vi "GetPositionDegreesSpeed.vi"(0 "StepMotor in":refnum<class "StepMotor.lvclass">, 2 "Редукция":dbl, 3 "Разрешение энкодера":dbl, 5 "error in (no error)":errorcluster) -> (14 "StepMotor out":refnum<class "StepMotor.lvclass">, 16 "Значение":dbl, 17 "+360 -360":bool, 18 "+ 0 -":bool, 19 "error out":errorcluster)   [LabVIEW 2010, in "StepMotor.lvclass"]
doc: "Подпрограмма получает значение энкодера СПШ и в зависимости от редукции и разрешения энкодера пересчитывает в градусы, диапазон значений энкодера варьируется от \"+\" к \"-\" значениям, это значит, что двигатель делает два оборота в левую сторону отрицательные значения и в правую сторону положительные значения. \n\n- Выходной параметр \"+ 0 -\" фиксирует переход от положительного диапазона к отрицательному диапазону или на оборот. \n\n- Выходной параметр \"+360 -360\" фиксирует состояния выхода значения энкодера за диапазон допустимый, как положительных значений, так и отрицательные значений, допустимый диапазон рассчитывается в зависимости от входных параметров \"Редукция\" и \"Разрешение энкодера\". Этот параметр необходим для обнуления внутренних переменных СПШ \"Текущая позиция\" и \"Заданная позиция\" функцией PCUR внутреннего ПЛК СПШ путём вызова из банка программ программу, в которой эта функция прописана\nПример:\n X=W //Сохраняем текущую скорость в переменную X\n W=0,A=10000 //Обнуляем скорость с ускорением 10000\n P=P,A=10000 // Заданной позиции присваиваем Текущую позицию\n PCUR=0 // Обнуляем текущую позицию и заданную позицию\n W=X // Присваиваем скорости значение сохранённое в переменной X\n HALT // Конец программы\n\nЭто позволяет контролировать много оборотов вала редуктора или двигателя при вращении в одну сторону, так как значение энкодера СПШ инкрементируются до ограниченного размера переменной в памяти контроллера ПЛК СПШ и ограничиваются диапазоном от 2147483648(параметр ПЛК ip14 прав.) до -2147483648(параметр ПЛК ip13 лев.) .\n\n-Выходной параметр \"Значение\" возвращает значение энкодера переведённое в градусы"
uses:
  StepMotor.lvclass
panel:
  out "Waveform Chart":dynamicdata(graph)
  out "РазностьТекущПреды":dbl
  out "RawValue":dbl
  out "МножПриведШкалы360":dbl
  out "КолИмпулОборот":dbl
  out "Текущая позиция":dbl
  out "Предыдущая позиция":dbl
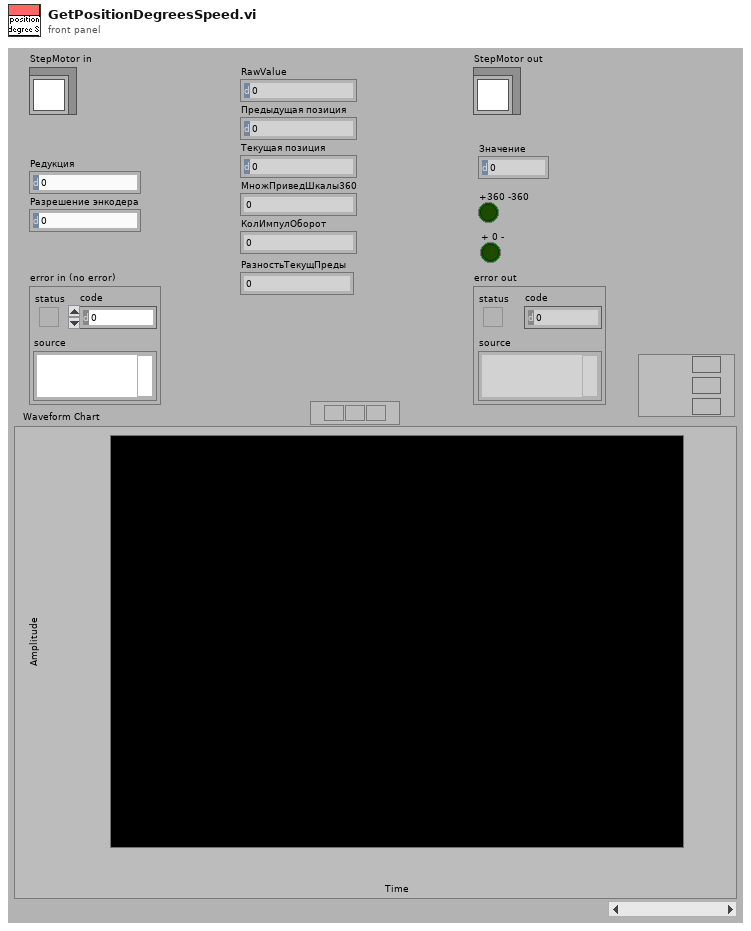
[diagram p1: front panel]
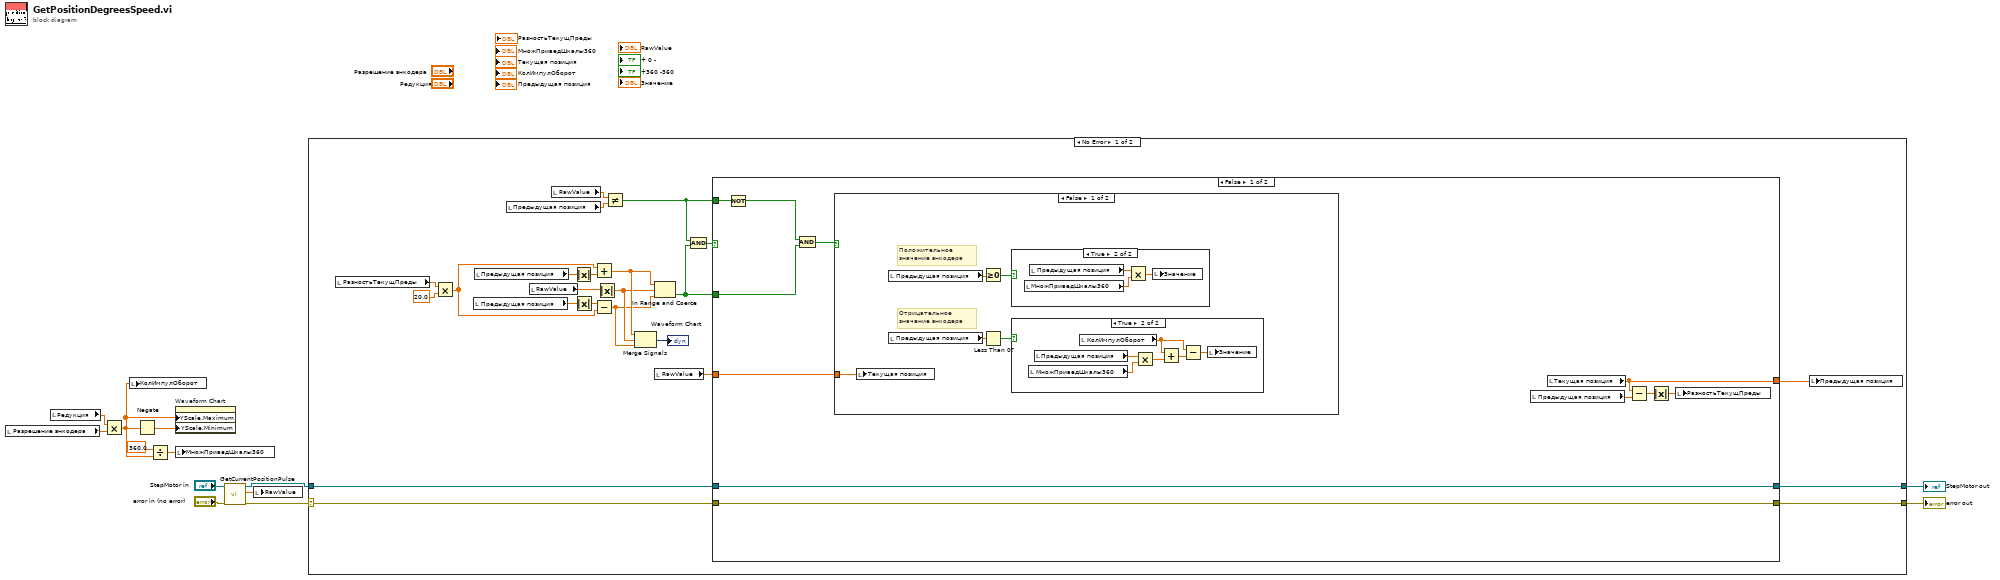
[diagram p0: block diagram]
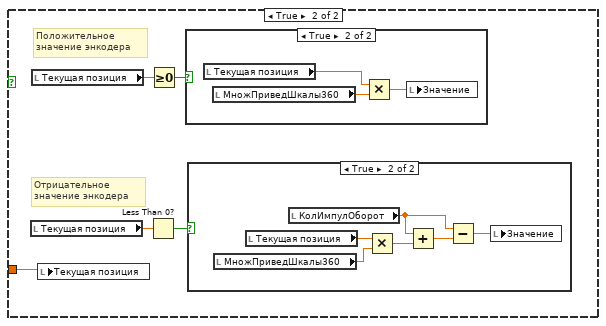
[diagram p4: hidden frame]
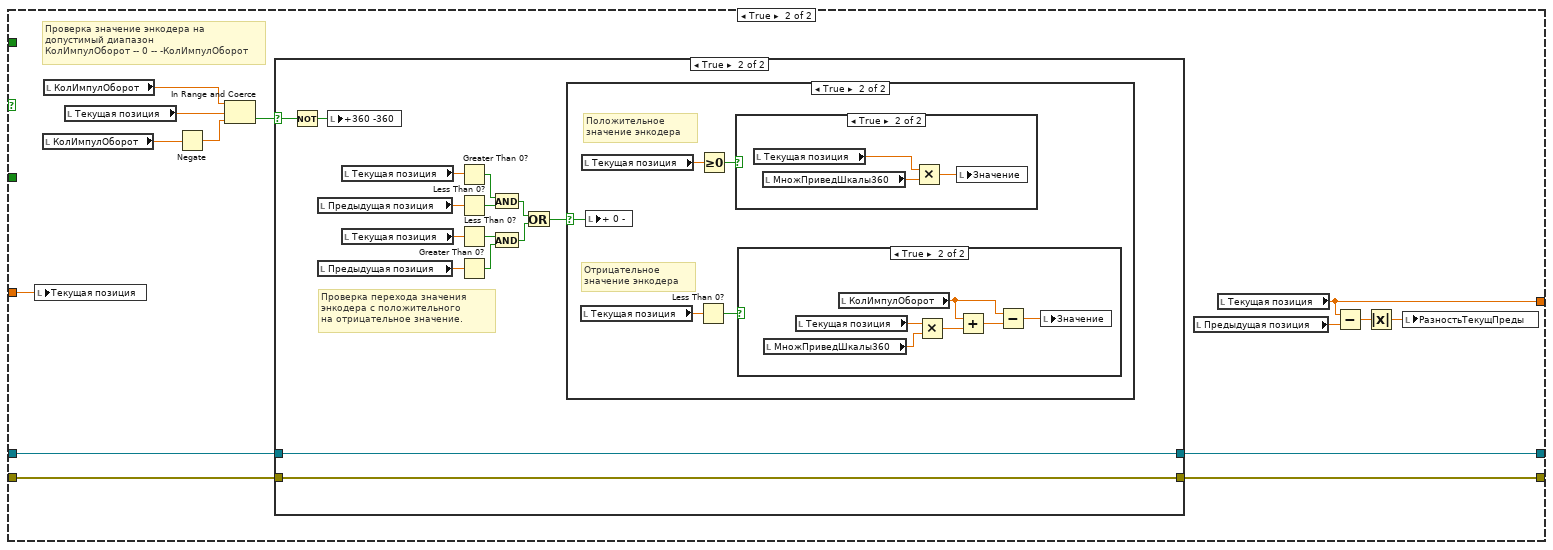
[diagram p7: hidden frame]
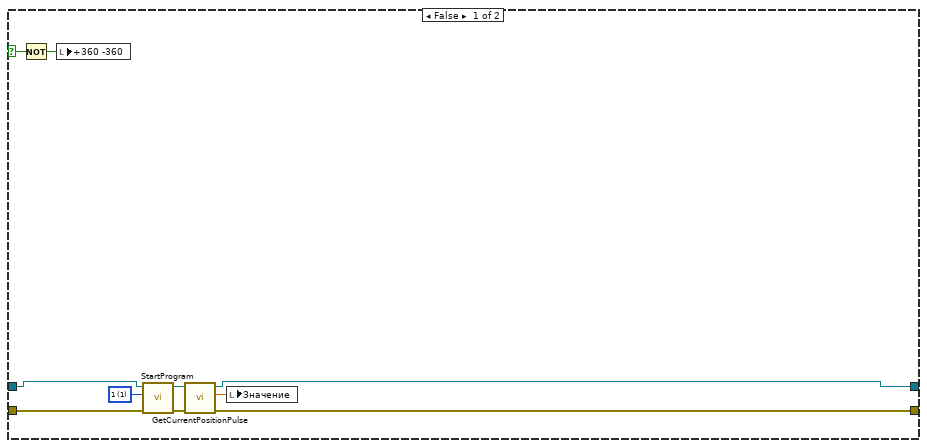
[diagram p8: hidden frame]
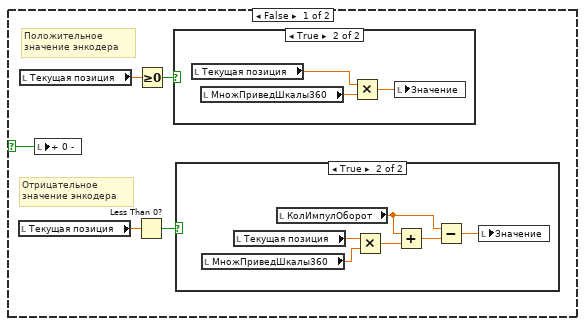
[diagram p9: hidden frame]
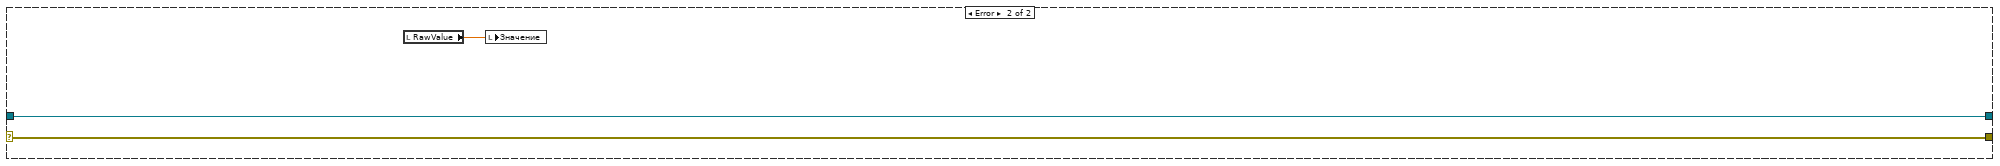
[diagram p14: hidden frame]
diagram:
  n1 = local read "Разрешение энкодера"() -> (w9:dbl)
  n2 = local read "Редукция"() -> (w8:dbl)
  n3 = Multiply(x=w8, y=w9) -> (x*y=w1:dbl)
  n4 = local write "КолИмпулОборот"(w1) -> ()
  n5 = Negate(x=w1) -> (-x=w2:dbl)
  n6 = Divide(x=360.0, y=w1) -> (x/y=w11:dbl)
  n7 = property on="Waveform Chart" class="WFChart (strict)"("YScale.Maximum"=w1, "YScale.Minimum"=w2) -> ()  [unwired: 2 in, 2 out]
  n8 = local write "МножПриведШкалы360"(w11) -> ()
  n9 = call-dynamic "GetCurrentPositionPulse.vi"("error in (no error)"="error in (no error)", "StepMotor in"="StepMotor in") -> ("error out"=w3:errorcluster, "Текущая позиция"=w7:dbl, "StepMotor out"=w4:refnum<class "StepMotor.lvclass">)  [unwired: 7 in]
  n10 = local write "RawValue"(w7) -> ()
  n11 = case shown="No Error" w3 {
    selector: w3 -> [w23 w144]
    tunnel: w4 -> [w24 w145]
    tunnel: [w36 w145] -> w12
    tunnel: [w35 w144] -> w13
    frame No Error {
      n12 = local read "РазностьТекущПреды"() -> (w19:dbl)
      n13 = Multiply(x=w19, y=20.0) -> (x*y=w26:dbl)
      n14 = local read "Предыдущая позиция"() -> (w29:dbl)
      n15 = local read "Предыдущая позиция"() -> (w27:dbl)
      n16 = local read "Предыдущая позиция"() -> (w34:dbl)
      n17 = local read "RawValue"() -> (w21:dbl)
      n18 = local read "RawValue"() -> (w22:dbl)
      n19 = Absolute Value(x=w27) -> (abs(x)=w30:dbl)
      n20 = Absolute Value(x=w29) -> (abs(x)=w28:dbl)
      n21 = Add(x=w26, y=w30) -> (x+y=w17:dbl)
      n22 = Subtract(x=w28, y=w26) -> (x-y=w15:dbl)
      n23 = Absolute Value(x=w21) -> (abs(x)=w16:dbl)
      n24 = Not Equal?(x=w22, y=w34) -> (x != y?=w31:bool)
      n25 = Merge Signals(w17, w16, w15) -> (→"Waveform Chart":dynamicdata)
      n26 = In Range and Coerce(upper limit=w17, x=w16, lower limit=w15) -> (In Range?=w32:bool)  [unwired: 1 out]
      n27 = local read "RawValue"() -> (w20:dbl)
      n28 = Compound Arithmetic op=AND(w31, w32) -> (w33:bool)
      n29 = case shown="False" w33 {
        tunnel: w32 -> [w42 _]
        tunnel: w31 -> [w45 _]
        tunnel: w24 -> [w47 w89]
        tunnel: w23 -> [w46 w88]
        tunnel: [w47 w87] -> w36
        tunnel: [w46 w86] -> w35
        tunnel: w20 -> [w41 w80]
        tunnel: [w37 w76] -> w18
        frame False {
          n30 = Not(x=w45) -> (.not. x?=w44:bool)
          n31 = Compound Arithmetic op=AND(w44, w42) -> (w43:bool)
          n32 = case shown="False" w43 {
            tunnel: w41 -> [w48 w62]
            frame False {
              # "Отрицательное \nзначение энкодера"
              # "Положительное \nзначение энкодера"
              n33 = local write "Текущая позиция"(w48) -> ()
              n34 = local read "Предыдущая позиция"() -> (w50:dbl)
              n35 = local read "Предыдущая позиция"() -> (w49:dbl)
              n36 = Greater Or Equal To 0?(x=w50) -> (x >= 0?=w52:bool)
              n37 = Less Than 0?(x=w49) -> (x < 0?=w51:bool)
              n38 = case shown="True" w52 {
                frame False {
                }
                frame True {
                  n39 = local read "МножПриведШкалы360"() -> (w61:dbl)
                  n40 = local read "Предыдущая позиция"() -> (w59:dbl)
                  n41 = Multiply(x=w59, y=w61) -> (x*y=w60:dbl)
                  n42 = local write "Значение"(w60) -> ()
                }
              }
              n43 = case shown="True" w51 {
                frame False {
                }
                frame True {
                  n44 = local read "МножПриведШкалы360"() -> (w58:dbl)
                  n45 = local read "Предыдущая позиция"() -> (w57:dbl)
                  n46 = local read "КолИмпулОборот"() -> (w55:dbl)
                  n47 = Multiply(x=w57, y=w58) -> (x*y=w56:dbl)
                  n48 = Add(x=w55, y=w56) -> (x+y=w54:dbl)
                  n49 = Subtract(x=w55, y=w54) -> (x-y=w53:dbl)
                  n50 = local write "Значение"(w53) -> ()
                }
              }
            }
            frame True {
              # "Отрицательное \nзначение энкодера"
              # "Положительное \nзначение энкодера"
              n51 = local read "Текущая позиция"() -> (w66:dbl)
              n52 = local read "Текущая позиция"() -> (w65:dbl)
              n53 = local write "Текущая позиция"(w62) -> ()
              n54 = Less Than 0?(x=w66) -> (x < 0?=w63:bool)
              n55 = Greater Or Equal To 0?(x=w65) -> (x >= 0?=w64:bool)
              n56 = case shown="True" w64 {
                frame False {
                }
                frame True {
                  n57 = local read "Текущая позиция"() -> (w73:dbl)
                  n58 = local read "МножПриведШкалы360"() -> (w75:dbl)
                  n59 = Multiply(x=w73, y=w75) -> (x*y=w74:dbl)
                  n60 = local write "Значение"(w74) -> ()
                }
              }
              n61 = case shown="True" w63 {
                frame False {
                }
                frame True {
                  n62 = local read "МножПриведШкалы360"() -> (w72:dbl)
                  n63 = local read "Текущая позиция"() -> (w71:dbl)
                  n64 = local read "КолИмпулОборот"() -> (w69:dbl)
                  n65 = Multiply(x=w71, y=w72) -> (x*y=w70:dbl)
                  n66 = Add(x=w69, y=w70) -> (x+y=w68:dbl)
                  n67 = Subtract(x=w69, y=w68) -> (x-y=w67:dbl)
                  n68 = local write "Значение"(w67) -> ()
                }
              }
            }
          }
          n69 = local read "Предыдущая позиция"() -> (w39:dbl)
          n70 = local read "Текущая позиция"() -> (w37:dbl)
          n71 = Subtract(x=w37, y=w39) -> (x-y=w40:dbl)
          n72 = Absolute Value(x=w40) -> (abs(x)=w38:dbl)
          n73 = local write "РазностьТекущПреды"(w38) -> ()
        }
        frame True {
          # "Проверка значение энкодера на\nдопустимый диапазон \nКолИмпулОборот -- 0 -- -КолИмпулОборот"
          n74 = local write "Текущая позиция"(w80) -> ()
          n75 = local read "КолИмпулОборот"() -> (w82:dbl)
          n76 = local read "КолИмпулОборот"() -> (w83:dbl)
          n77 = local read "Текущая позиция"() -> (w81:dbl)
          n78 = Negate(x=w82) -> (-x=w85:dbl)
          n79 = In Range and Coerce(upper limit=w83, x=w81, lower limit=w85) -> (In Range?=w84:bool)  [unwired: 1 out]
          n80 = case shown="True" w84 {
            selector: w84 -> [w96 w100]
            tunnel: w89 -> [w93 w103]
            tunnel: w88 -> [w92 w102]
            tunnel: [w98 w103] -> w87
            tunnel: [w97 w102] -> w86
            frame False {
              w99 = u16 1 items=["0", "1", "2", "3", "4", "5", "6", "7"] ("Номер банка программ")
              n81 = Not(x=w96) -> (.not. x?=w95:bool)
              n82 = local write "+360 -360"(w95) -> ()
              n83 = call-dynamic "StartProgram.vi"("error in (no error)"=w92, "Номер банка программ"=w99, "StepMotor in"=w93) -> ("error out"=w90:errorcluster, "StepMotor out"=w91:refnum<class "StepMotor.lvclass">)  [unwired: 7 in]
              n84 = call-dynamic "GetCurrentPositionPulse.vi"("error in (no error)"=w90, "StepMotor in"=w91) -> ("error out"=w97:errorcluster, "Текущая позиция"=w94:dbl, "StepMotor out"=w98:refnum<class "StepMotor.lvclass">)  [unwired: 7 in]
              n85 = local write "Значение"(w94) -> ()
            }
            frame True {
              # "Проверка перехода значения \nэнкодера с положительного\nна отрицательное значение."
              n86 = Not(x=w100) -> (.not. x?=w101:bool)
              n87 = local read "Предыдущая позиция"() -> (w105:dbl)
              n88 = local read "Предыдущая позиция"() -> (w104:dbl)
              n89 = local write "+360 -360"(w101) -> ()
              n90 = local read "Текущая позиция"() -> (w107:dbl)
              n91 = local read "Текущая позиция"() -> (w106:dbl)
              n92 = Greater Than 0?(x=w107) -> (x > 0?=w110:bool)
              n93 = Less Than 0?(x=w105) -> (x < 0?=w111:bool)
              n94 = Less Than 0?(x=w106) -> (x < 0?=w109:bool)
              n95 = Greater Than 0?(x=w104) -> (x > 0?=w108:bool)
              n96 = And(x=w110, y=w111) -> (x .and. y?=w112:bool)
              n97 = And(x=w109, y=w108) -> (x .and. y?=w113:bool)
              n98 = Or(x=w112, y=w113) -> (x .or. y?=w114:bool)
              n99 = case shown="True" w114 {
                selector: w114 -> [w115 w129]
                frame False {
                  # "Отрицательное \nзначение энкодера"
                  # "Положительное \nзначение энкодера"
                  n100 = local read "Текущая позиция"() -> (w119:dbl)
                  n101 = local read "Текущая позиция"() -> (w118:dbl)
                  n102 = local write "+ 0 -"(w115) -> ()
                  n103 = Less Than 0?(x=w119) -> (x < 0?=w116:bool)
                  n104 = Greater Or Equal To 0?(x=w118) -> (x >= 0?=w117:bool)
                  n105 = case shown="True" w117 {
                    frame False {
                    }
                    frame True {
                      n106 = local read "Текущая позиция"() -> (w126:dbl)
                      n107 = local read "МножПриведШкалы360"() -> (w128:dbl)
                      n108 = Multiply(x=w126, y=w128) -> (x*y=w127:dbl)
                      n109 = local write "Значение"(w127) -> ()
                    }
                  }
                  n110 = case shown="True" w116 {
                    frame False {
                    }
                    frame True {
                      n111 = local read "МножПриведШкалы360"() -> (w125:dbl)
                      n112 = local read "Текущая позиция"() -> (w124:dbl)
                      n113 = local read "КолИмпулОборот"() -> (w122:dbl)
                      n114 = Multiply(x=w124, y=w125) -> (x*y=w123:dbl)
                      n115 = Add(x=w122, y=w123) -> (x+y=w121:dbl)
                      n116 = Subtract(x=w122, y=w121) -> (x-y=w120:dbl)
                      n117 = local write "Значение"(w120) -> ()
                    }
                  }
                }
                frame True {
                  # "Отрицательное \nзначение энкодера"
                  # "Положительное \nзначение энкодера"
                  n118 = local read "Текущая позиция"() -> (w133:dbl)
                  n119 = local read "Текущая позиция"() -> (w132:dbl)
                  n120 = local write "+ 0 -"(w129) -> ()
                  n121 = Less Than 0?(x=w133) -> (x < 0?=w130:bool)
                  n122 = Greater Or Equal To 0?(x=w132) -> (x >= 0?=w131:bool)
                  n123 = case shown="True" w131 {
                    frame False {
                    }
                    frame True {
                      n124 = local read "Текущая позиция"() -> (w140:dbl)
                      n125 = local read "МножПриведШкалы360"() -> (w142:dbl)
                      n126 = Multiply(x=w140, y=w142) -> (x*y=w141:dbl)
                      n127 = local write "Значение"(w141) -> ()
                    }
                  }
                  n128 = case shown="True" w130 {
                    frame False {
                    }
                    frame True {
                      n129 = local read "МножПриведШкалы360"() -> (w139:dbl)
                      n130 = local read "Текущая позиция"() -> (w138:dbl)
                      n131 = local read "КолИмпулОборот"() -> (w136:dbl)
                      n132 = Multiply(x=w138, y=w139) -> (x*y=w137:dbl)
                      n133 = Add(x=w136, y=w137) -> (x+y=w135:dbl)
                      n134 = Subtract(x=w136, y=w135) -> (x-y=w134:dbl)
                      n135 = local write "Значение"(w134) -> ()
                    }
                  }
                }
              }
            }
          }
          n136 = local read "Предыдущая позиция"() -> (w78:dbl)
          n137 = local read "Текущая позиция"() -> (w76:dbl)
          n138 = Subtract(x=w76, y=w78) -> (x-y=w79:dbl)
          n139 = Absolute Value(x=w79) -> (abs(x)=w77:dbl)
          n140 = local write "РазностьТекущПреды"(w77) -> ()
        }
      }
      n141 = local write "Предыдущая позиция"(w18) -> ()
    }
    frame Error {
      n142 = local read "RawValue"() -> (w143:dbl)
      n143 = local write "Значение"(w143) -> ()
    }
  }
  "error out" <- w13
  "StepMotor out" <- w12
